vi "Format number_1234567890.vi"(1 "number":dbl=1445234.0 format="%#_6p") -> (0 "String":string)   [LabVIEW 2011]
panel:
  in  "length":i32=13
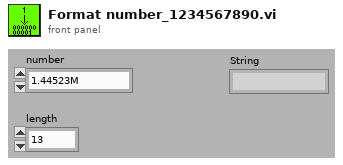
[diagram p1: front panel]
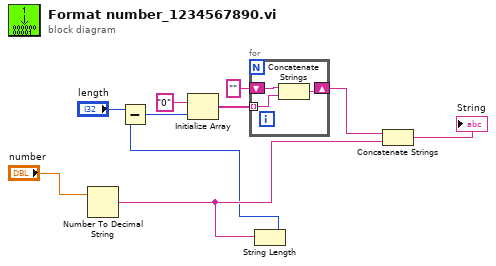
[diagram p0: block diagram]
diagram:
  n1 = Number To Decimal String(number="number") -> (decimal integer string=w9:string)  [unwired: 1 out]
  n2 = String Length(string=w9) -> (length=w3:i32)
  n3 = Subtract(x="length", y=w3) -> (x-y=w4:i32)
  n4 = Initialize Array("0" ("string"), w4) -> (w7:string[])
  n5 = for {
    tunnel: w7 -> [w13] mode=indexing
    shift-right: [w12] -> w5
    shift-left: "" -> [w11]
    n6 = Concatenate Strings(w11, w13) -> (w12:string)
  }
  n7 = Concatenate Strings(w5, w9) -> (→"String":string)
